vi "CRYMultimeter Scale Change.vi"(5 "Limits":u16(ring)=2 items=["Upper Only", "Lower Only", "Upper & Lower"], 6 "Multi Val":dbl format="%#.3p", 7 "Single Limit":refnum<vi>, 8 "Low Limit":dbl, 9 "Up Limit":dbl, 10 "Multi value":refnum<vi>, 11 "Multi limit":refnum<vi>) -> (2 "Lo tip":cluster{dbl, dbl}, 3 "Up tip":cluster{dbl, dbl})   [LabVIEW 2013]
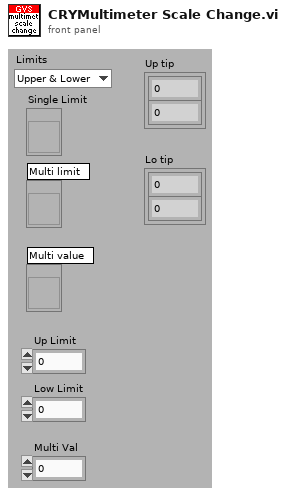
[diagram p1: front panel]
types:
  T1 = typedef "LVPositionTypeDef.ctl" = cluster{"Left":i32, "Top":i32}
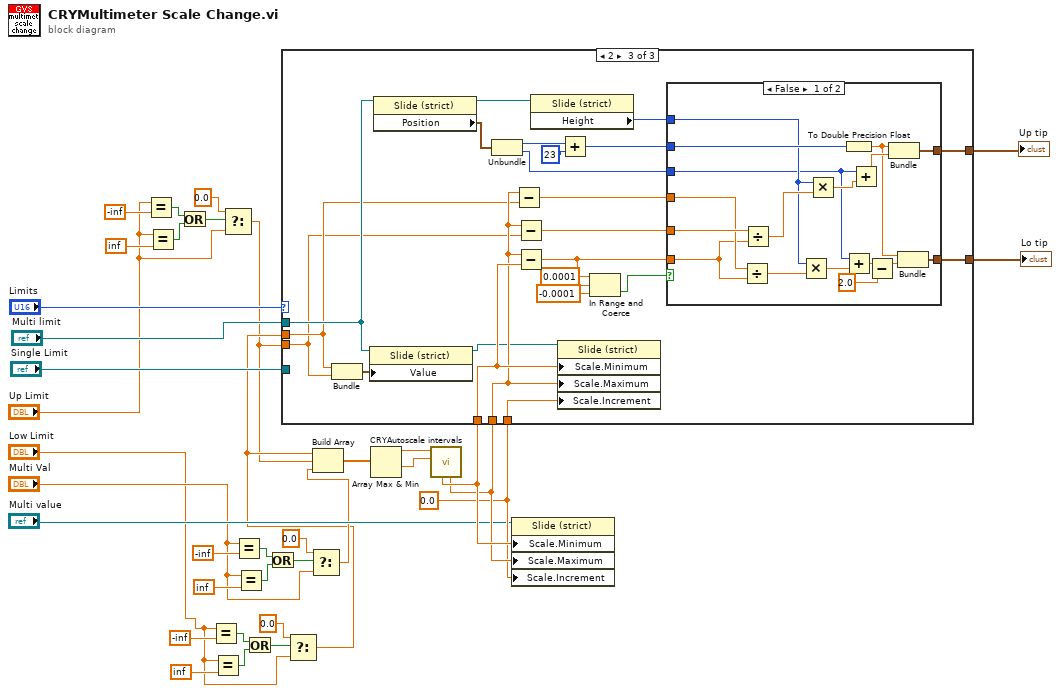
[diagram p0: block diagram]
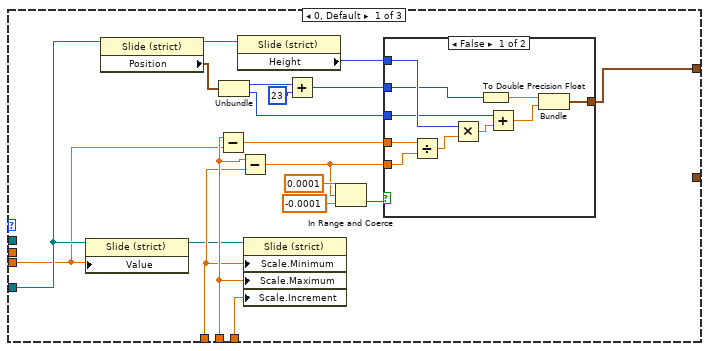
[diagram p2: hidden frame]
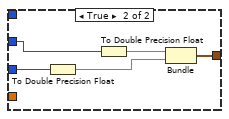
[diagram p3: hidden frame]
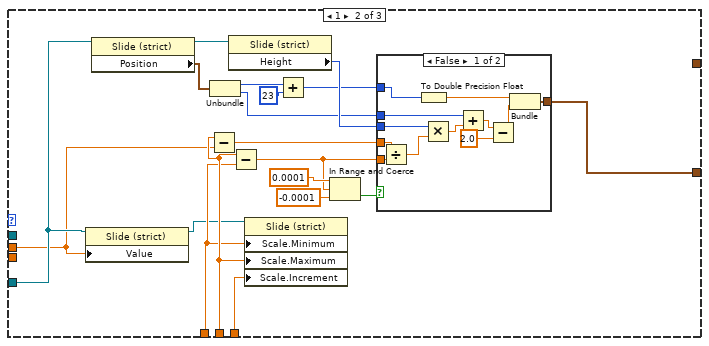
[diagram p4: hidden frame]
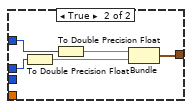
[diagram p5: hidden frame]
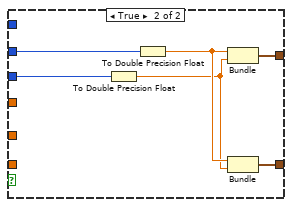
[diagram p6: hidden frame]
diagram:
  w30 = 0.0
  n1 = Equal?(x="Up Limit", y=-inf) -> (x = y?=w6:bool)
  n2 = Equal?(x="Up Limit", y=inf) -> (x = y?=w5:bool)
  n3 = Or(x=w6, y=w5) -> (x .or. y?=w4:bool)
  n4 = Equal?(x="Low Limit", y=-inf) -> (x = y?=w13:bool)
  n5 = Equal?(x="Low Limit", y=inf) -> (x = y?=w14:bool)
  n6 = Select(t=0.0, s=w4, f="Up Limit") -> (s? t:f=w1:dbl)
  n7 = Equal?(x="Multi Val", y=-inf) -> (x = y?=w22:bool)
  n8 = Equal?(x="Multi Val", y=inf) -> (x = y?=w21:bool)
  n9 = Or(x=w13, y=w14) -> (x .or. y?=w15:bool)
  n10 = Or(x=w22, y=w21) -> (x .or. y?=w20:bool)
  n11 = Select(t=0.0, s=w15, f="Low Limit") -> (s? t:f=w9:dbl)
  n12 = Select(t=0.0, s=w20, f="Multi Val") -> (s? t:f=w17:dbl)
  n13 = Build Array(w9, w1, w17) -> (w36:dbl[])
  n14 = Array Max & Min(array=w36) -> (max value=w35:dbl, min value=w34:dbl)  [unwired: 2 out]
  n15 = call "CRYAutoscale intervals.vi"("Minimum value (0.0)"=w34, "Maximum value"=w35) -> ("Scale max."=w31:dbl, "Scale min."=w32:dbl)  [unwired: 2 in, 6 out]
  n16 = case shown="2" "Limits" {
    tunnel: "Multi limit" -> [_ _ w117]
    tunnel: w1 -> [w42 _ w113]
    tunnel: w9 -> [_ w77 w114]
    tunnel: w32 -> [w52 w79 w128]
    tunnel: w31 -> [w53 w80 w118]
    tunnel: w30 -> [w55 w89 w129]
    tunnel: "Single Limit" -> [w44 w78 _]
    tunnel: [w37 _ w108] -> w26
    tunnel: [_ w71 w107] -> w25
    frame 0, Default {
      n17 = property class="Slide (strict)"(reference=w44, "Value"=w42) -> (reference out=w43:refnum<vi>)  [unwired: 1 in, 1 out]
      n18 = property class="Slide (strict)"(reference=w44) -> (reference out=w54:refnum<vi>, "Position"=w49:T1)  [unwired: 1 in, 1 out]
      n19 = Subtract(x=w53, y=w42) -> (x-y=w51:dbl)
      n20 = Unbundle(w49) -> ("Left"=w48:i32, "Top"=w46:i32)
      n21 = property class="Slide (strict)"(reference=w54) -> ("Height"=w50:u32)  [unwired: 1 in, 2 out]
      n22 = Subtract(x=w53, y=w52) -> (x-y=w39:dbl)
      n23 = property class="Slide (strict)"(reference=w43, "Scale.Minimum"=w52, "Scale.Maximum"=w53, "Scale.Increment"=w55) -> ()  [unwired: 1 in, 2 out]
      n24 = Add(x=w48, y=23) -> (x+y=w45:i32)
      n25 = In Range and Coerce(upper limit=0.0001, x=w39, lower limit=-0.0001) -> (In Range?=w38:bool)  [unwired: 1 out]
      n26 = case shown="False" w38 {
        tunnel: w51 -> [w65 _]
        tunnel: w50 -> [w63 _]
        tunnel: w46 -> [w60 w67]
        tunnel: w45 -> [w59 w69]
        tunnel: [w57 w70] -> w37
        tunnel: w39 -> [w56 _]
        frame False {
          n27 = Divide(x=w65, y=w56) -> (x/y=w64:dbl)
          n28 = Multiply(x=w63, y=w64) -> (x*y=w61:dbl)
          n29 = To Double Precision Float(number=w59) -> (double precision float=w58:dbl)
          n30 = Add(x=w60, y=w61) -> (x+y=w62:dbl)
          n31 = Bundle(w58, w62) -> (w57:cluster{dbl, dbl})  [unwired: 1 out]
        }
        frame True {
          n32 = To Double Precision Float(number=w67) -> (double precision float=w66:dbl)
          n33 = To Double Precision Float(number=w69) -> (double precision float=w68:dbl)
          n34 = Bundle(w68, w66) -> (w70:cluster{dbl, dbl})  [unwired: 1 out]
        }
      }
    }
    frame 1 {
      n35 = property class="Slide (strict)"(reference=w78, "Value"=w77) -> (reference out=w76:refnum<vi>)  [unwired: 1 in, 1 out]
      n36 = property class="Slide (strict)"(reference=w78) -> (reference out=w88:refnum<vi>, "Position"=w85:T1)  [unwired: 1 in, 1 out]
      n37 = Subtract(x=w80, y=w77) -> (x-y=w87:dbl)
      n38 = Unbundle(w85) -> ("Left"=w84:i32, "Top"=w82:i32)
      n39 = property class="Slide (strict)"(reference=w88) -> ("Height"=w86:u32)  [unwired: 1 in, 2 out]
      n40 = Subtract(x=w80, y=w79) -> (x-y=w73:dbl)
      n41 = property class="Slide (strict)"(reference=w76, "Scale.Minimum"=w79, "Scale.Maximum"=w80, "Scale.Increment"=w89) -> ()  [unwired: 1 in, 2 out]
      n42 = Add(x=w84, y=23) -> (x+y=w81:i32)
      n43 = In Range and Coerce(upper limit=0.0001, x=w73, lower limit=-0.0001) -> (In Range?=w72:bool)  [unwired: 1 out]
      n44 = case shown="False" w72 {
        tunnel: w87 -> [w101 _]
        tunnel: w86 -> [w99 _]
        tunnel: w82 -> [w97 w105]
        tunnel: w81 -> [w96 w106]
        tunnel: [w94 w104] -> w71
        tunnel: w73 -> [w93 _]
        frame False {
          n45 = Divide(x=w101, y=w93) -> (x/y=w100:dbl)
          n46 = To Double Precision Float(number=w96) -> (double precision float=w95:dbl)
          n47 = Multiply(x=w99, y=w100) -> (x*y=w98:dbl)
          n48 = Add(x=w97, y=w98) -> (x+y=w91:dbl)
          n49 = Subtract(x=w91, y=2.0) -> (x-y=w92:dbl)
          n50 = Bundle(w95, w92) -> (w94:cluster{dbl, dbl})  [unwired: 1 out]
        }
        frame True {
          n51 = To Double Precision Float(number=w105) -> (double precision float=w102:dbl)
          n52 = To Double Precision Float(number=w106) -> (double precision float=w103:dbl)
          n53 = Bundle(w103, w102) -> (w104:cluster{dbl, dbl})  [unwired: 1 out]
        }
      }
    }
    frame 2 {
      n54 = Bundle("Low Limit"=w114, "Up Limit"=w113) -> (w115:cluster{"Low Limit":dbl, "Up Limit":dbl})  [unwired: 1 out]
      n55 = property class="Slide (strict)"(reference=w117, "Value"=w115) -> (reference out=w116:refnum<vi>)  [unwired: 1 in, 1 out]
      n56 = property class="Slide (strict)"(reference=w117) -> (reference out=w127:refnum<vi>, "Position"=w125:T1)  [unwired: 1 in, 1 out]
      n57 = Unbundle(w125) -> ("Left"=w124:i32, "Top"=w119:i32)
      n58 = Subtract(x=w118, y=w114) -> (x-y=w121:dbl)
      n59 = Subtract(x=w118, y=w113) -> (x-y=w126:dbl)
      n60 = Subtract(x=w118, y=w128) -> (x-y=w112:dbl)
      n61 = property class="Slide (strict)"(reference=w127) -> ("Height"=w120:u32)  [unwired: 1 in, 2 out]
      n62 = property class="Slide (strict)"(reference=w116, "Scale.Minimum"=w128, "Scale.Maximum"=w118, "Scale.Increment"=w129) -> ()  [unwired: 1 in, 2 out]
      n63 = Add(x=w124, y=23) -> (x+y=w122:i32)
      n64 = In Range and Coerce(upper limit=0.0001, x=w112, lower limit=-0.0001) -> (In Range?=w109:bool)  [unwired: 1 out]
      n65 = case shown="False" w109 {
        tunnel: w126 -> [w146 _]
        tunnel: w122 -> [w143 w152]
        tunnel: w121 -> [w141 _]
        tunnel: w120 -> [w139 _]
        tunnel: w119 -> [w137 w150]
        tunnel: [w134 w148] -> w108
        tunnel: [w133 w147] -> w107
        tunnel: w112 -> [w132 _]
        frame False {
          n66 = Divide(x=w141, y=w132) -> (x/y=w140:dbl)
          n67 = Divide(x=w146, y=w132) -> (x/y=w145:dbl)
          n68 = Multiply(x=w139, y=w140) -> (x*y=w138:dbl)
          n69 = Multiply(x=w139, y=w145) -> (x*y=w142:dbl)
          n70 = To Double Precision Float(number=w143) -> (double precision float=w135:dbl)
          n71 = Add(x=w137, y=w138) -> (x+y=w136:dbl)
          n72 = Add(x=w137, y=w142) -> (x+y=w144:dbl)
          n73 = Subtract(x=w136, y=2.0) -> (x-y=w131:dbl)
          n74 = Bundle(w135, w144) -> (w134:cluster{dbl, dbl})  [unwired: 1 out]
          n75 = Bundle(w135, w131) -> (w133:cluster{dbl, dbl})  [unwired: 1 out]
        }
        frame True {
          n76 = To Double Precision Float(number=w150) -> (double precision float=w149:dbl)
          n77 = To Double Precision Float(number=w152) -> (double precision float=w151:dbl)
          n78 = Bundle(w151, w149) -> (w148:cluster{dbl, dbl})  [unwired: 1 out]
          n79 = Bundle(w151, w149) -> (w147:cluster{dbl, dbl})  [unwired: 1 out]
        }
      }
    }
  }
  "Up tip" <- w26
  "Lo tip" <- w25
  n80 = property class="Slide (strict)"(reference="Multi value", "Scale.Minimum"=w32, "Scale.Maximum"=w31, "Scale.Increment"=w30) -> ()  [unwired: 1 in, 2 out]
